vi "AMLUTwaveselHD2.vi"(0 "AM Freq Hz":dbl=1000.0, 5 "Peak Power":dbl=20.0, 7 "Min Power":dbl=10.0, 9 "Wave Shape":u8(ring) items=["Sine", "Ramp", "Triangle"], 11 "HD2?":bool, 12 "Linear in?":u8(ring) items=["Linear in dB", "Linear in Volts"]) -> (4 "Waveform":dbl[](graph), 8 "Actual Freq":dbl=1000.0, 13 "LUTsize":u8=32, 15 "powerout":string)   [LabVIEW 2017]
panel:
  out "stdam":u16
  # "dBm"
  # "dBm"
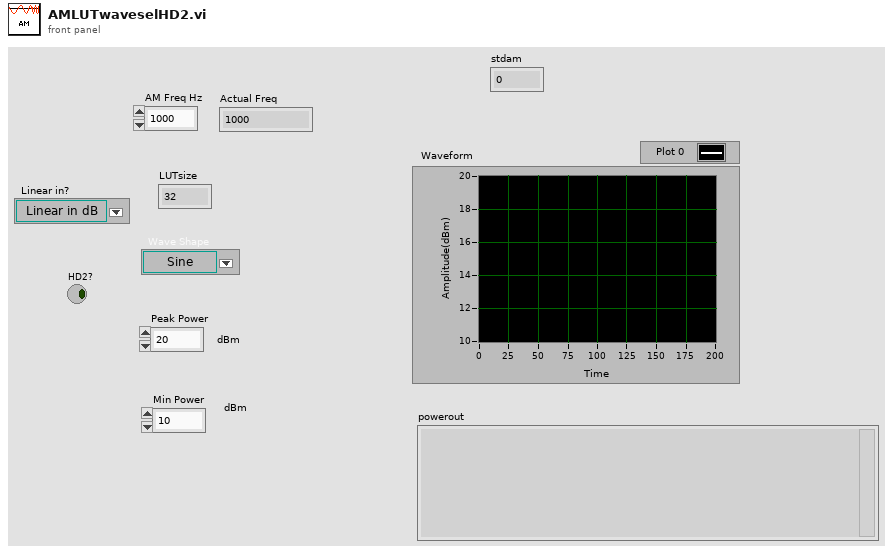
[diagram p1: front panel]
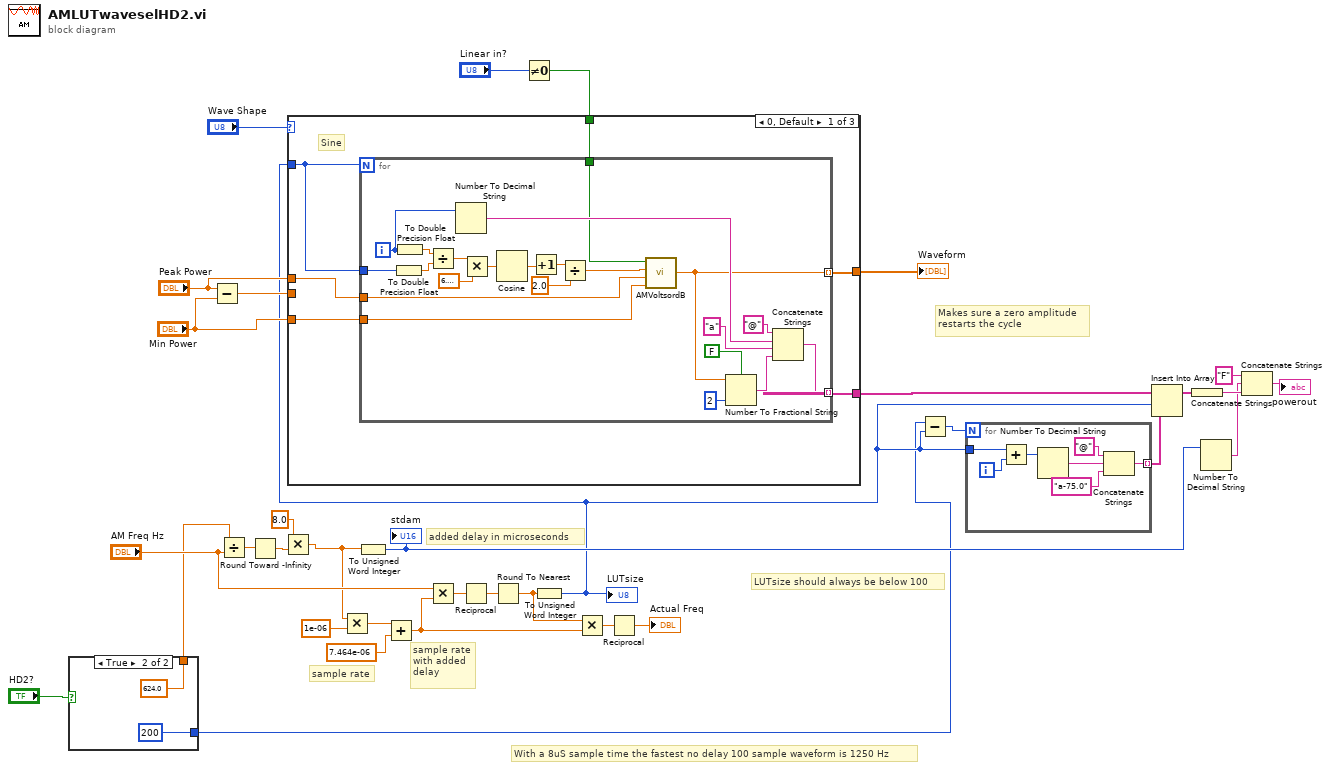
[diagram p0: block diagram]
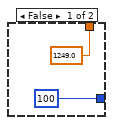
[diagram p2: hidden frame]
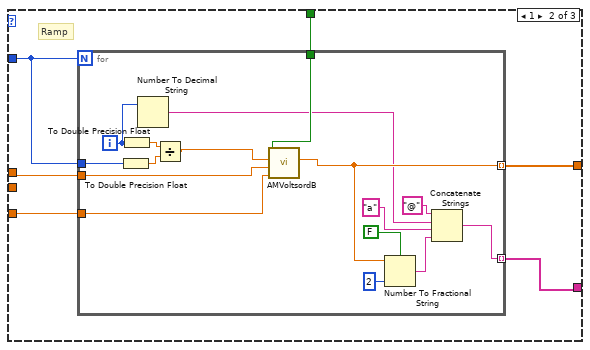
[diagram p3: hidden frame]
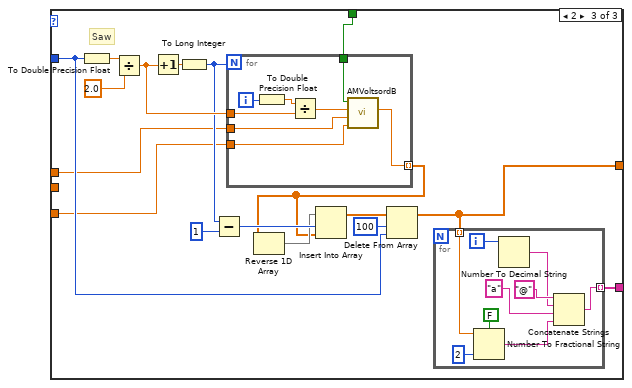
[diagram p4: hidden frame]
diagram:
  # "With a 8uS sample time the fastest no delay 100 sample waveform is 1250 Hz"
  # "LUTsize should always be below 100"
  # "added delay in microseconds"
  # "sample rate\nwith added\ndelay"
  # "sample rate"
  # "Makes sure a zero amplitude\nrestarts the cycle"
  n1 = case shown="True" "HD2?" {
    tunnel: [u8 100 ("y") u8 200 ("y")] -> w2
    tunnel: [1249.0 ("x") 624.0 ("x")] -> w1
    frame False {
    }
    frame True {
    }
  }
  n2 = Subtract(x="Peak Power", y="Min Power") -> (x-y=w33:dbl)
  n3 = Divide(x=w1, y="AM Freq Hz") -> (x/y=w13:dbl)
  n4 = Round Toward -Infinity(1:w13) -> (0:w12:dbl)
  n5 = Multiply(x=8.0, y=w12) -> (x*y=w11:dbl)
  n6 = Multiply(x=w11, y=1e-06) -> (x*y=w23:dbl)
  n7 = To Unsigned Word Integer(number=w11) -> (unsigned 16bit integer=w26:u16)
  "stdam" <- w26
  n8 = Add(x=w23, y=7.464e-06 ("x")) -> (x+y=w15:dbl)
  n9 = Multiply(x="AM Freq Hz", y=w15) -> (x*y=w21:dbl)
  n10 = Reciprocal(x=w21) -> (1/x=w20:dbl)
  n11 = Round To Nearest(number=w20) -> (nearest integer value=w16:dbl)
  n12 = Not Equal To 0?(x="Linear in?") -> (x != 0?=w7:bool)
  n13 = To Unsigned Word Integer(number=w16) -> (unsigned 16bit integer=w5:u16)
  "LUTsize" <- w5
  n14 = case shown="0, Default" "Wave Shape" {
    tunnel: [w43 w72 w94] -> w9
    tunnel: w5 -> [w44 w71 w97]
    tunnel: "Min Power" -> [w42 w70 w95]
    tunnel: [w41 w69 w93] -> w31
    tunnel: w33 -> [_ _ _]
    tunnel: w7 -> [w40 w68 w91]
    tunnel: "Peak Power" -> [w39 w67 w92]
    frame 0, Default {
      # "Sine"
      n15 = for {
        N: w44 -> [_]
        tunnel: [w47] -> w43 mode=indexing
        tunnel: w44 -> [w61]
        tunnel: w42 -> [w54]
        tunnel: [w57] -> w41 mode=indexing
        tunnel: w40 -> [w56]
        tunnel: w39 -> [w55]
        i -> [w60]
        n16 = To Double Precision Float(number=w61) -> (double precision float=w62:dbl)
        n17 = To Double Precision Float(number=w60) -> (double precision float=w63:dbl)
        n18 = Divide(x=w63, y=w62) -> (x/y=w66:dbl)
        n19 = Number To Decimal String(number=w60) -> (decimal integer string=w59:string)  [unwired: 1 in]
        n20 = Multiply(x=w66, y=6.283185307179586) -> (x*y=w64:dbl)
        n21 = Cosine(x=w64) -> (cos(x)=w53:dbl)
        n22 = Increment(x=w53) -> (x+1=w52:dbl)
        n23 = Divide(x=w52, y=2.0) -> (x/y=w50:dbl)
        n24 = call "AMVoltsordB.vi"("Min Power"=w54, "Peak Power"=w55, "Signal In"=w50, "Linear?"=w56) -> ("Out"=w47:dbl)  [unwired: 7 in]
        n25 = Number To Fractional String(use system decimal point (T)=FALSE, number=w47, precision (6)=i16 2) -> (F-format string=w48:string)  [unwired: 1 in]
        n26 = Concatenate Strings("@" ("string"), w59, "a" ("string"), w48) -> (w57:string)
      }
    }
    frame 1 {
      # "Ramp"
      n27 = for {
        N: w71 -> [_]
        tunnel: [w75] -> w72 mode=indexing
        tunnel: w71 -> [w86]
        tunnel: w67 -> [w83]
        tunnel: w70 -> [w84]
        tunnel: [w73] -> w69 mode=indexing
        tunnel: w68 -> [w82]
        i -> [w85]
        n28 = To Double Precision Float(number=w86) -> (double precision float=w87:dbl)
        n29 = To Double Precision Float(number=w85) -> (double precision float=w88:dbl)
        n30 = Number To Decimal String(number=w85) -> (decimal integer string=w74:string)  [unwired: 1 in]
        n31 = Divide(x=w88, y=w87) -> (x/y=w81:dbl)
        n32 = call "AMVoltsordB.vi"("Min Power"=w84, "Peak Power"=w83, "Signal In"=w81, "Linear?"=w82) -> ("Out"=w75:dbl)  [unwired: 7 in]
        n33 = Number To Fractional String(use system decimal point (T)=FALSE, number=w75, precision (6)=i16 2) -> (F-format string=w78:string)  [unwired: 1 in]
        n34 = Concatenate Strings("@" ("string"), w74, "a" ("string"), w78) -> (w73:string)
      }
    }
    frame 2 {
      # "Saw"
      n35 = To Double Precision Float(number=w97) -> (double precision float=w105:dbl)
      n36 = Divide(x=w105, y=2.0) -> (x/y=w102:dbl)
      n37 = Increment(x=w102) -> (x+1=w103:dbl)
      n38 = To Long Integer(number=w103) -> (32bit integer=w101:i32)
      n39 = Subtract(x=w101, y=1) -> (x-y=w100:i32)
      n40 = for {
        N: w101 -> [_]
        tunnel: [w115] -> w89 mode=indexing
        tunnel: w102 -> [w120]
        tunnel: w92 -> [w117]
        tunnel: w95 -> [w118]
        tunnel: w91 -> [w116]
        i -> [w121]
        n41 = To Double Precision Float(number=w121) -> (double precision float=w122:dbl)
        n42 = Divide(x=w122, y=w120) -> (x/y=w119:dbl)
        n43 = call "AMVoltsordB.vi"("Min Power"=w118, "Peak Power"=w117, "Signal In"=w119, "Linear?"=w116) -> ("Out"=w115:dbl)  [unwired: 7 in]
      }
      n44 = Reverse 1D Array(array=w89) -> (reversed array=w90:dbl[])
      n45 = Insert Into Array(array=w90, index=w100, new element=w89) -> (w98:dbl[])
      n46 = Delete From Array(array=w98, length=100, index=w97) -> (array with subset deleted=w94:dbl[])  [unwired: 1 out]
      n47 = for {
        tunnel: w94 -> [w107] mode=indexing
        tunnel: [w112] -> w93 mode=indexing
        i -> [w114]
        n48 = Number To Fractional String(use system decimal point (T)=FALSE, number=w107, precision (6)=i16 2) -> (F-format string=w106:string)  [unwired: 1 in]
        n49 = Number To Decimal String(number=w114) -> (decimal integer string=w111:string)  [unwired: 1 in]
        n50 = Concatenate Strings("@" ("string"), w111, "a" ("string"), w106) -> (w112:string)
      }
    }
  }
  "Waveform" <- w9
  n51 = Multiply(x=w16, y=w15) -> (x*y=w19:dbl)
  n52 = Reciprocal(x=w19) -> (1/x=→"Actual Freq":dbl)
  n53 = Subtract(x=w2, y=w5) -> (x-y=w4:u16)
  n54 = for {
    N: w4 -> [_]
    tunnel: [w124] -> w6 mode=indexing
    tunnel: w5 -> [w123]
    i -> [w129]
    n55 = Add(x=w123, y=w129) -> (x+y=w125:i32)
    n56 = Number To Decimal String(number=w125) -> (decimal integer string=w127:string)  [unwired: 1 in]
    n57 = Concatenate Strings("@" ("string"), w127, "a-75.0" ("new element/subarray")) -> (w124:string)
  }
  n58 = Insert Into Array(array=w31, index=w5, new element=w6) -> (w30:string[])
  n59 = Concatenate Strings(w30) -> (w28:string)
  n60 = Number To Decimal String(number=w26) -> (decimal integer string=w27:string)  [unwired: 1 in]
  n61 = Concatenate Strings("F" ("string"), w27, w28) -> (→"powerout":string)
